vi "MH_BuffAndQDeltas.vi"(6 "queue out":refnum<queue>, 7 "DeltasBuffer":i32[](array[numeric]), 8 "erroIn":errorcluster caption="error In", 9 "WriteDelta":bool, 11 "Deltaindex":i32) -> (0 "error out":errorcluster, 1 "DeltaIndexOut":i32, 2 "DeltasBufferOut":i32[](array[numeric]))   [LabVIEW 2019]
uses:
  <userlib>/MultiHarp150/T2Lib/MH_T2DeltaQMessage.ctl
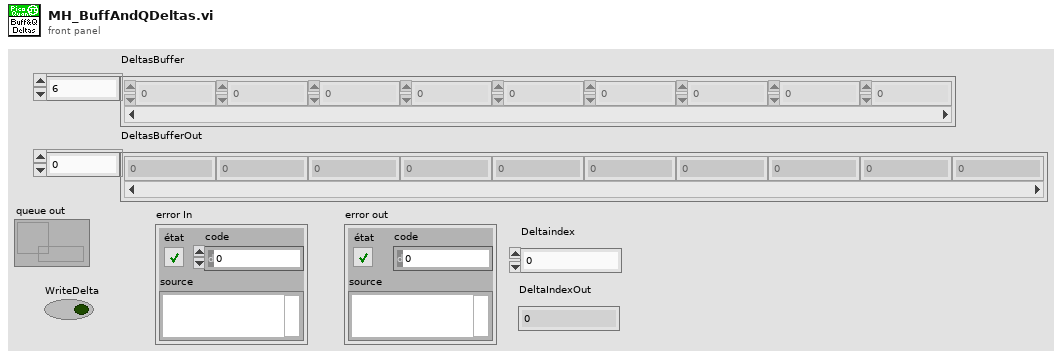
[diagram p1: front panel]
types:
  T1 = typedef "MH_T2DeltaQMessage.ctl" = cluster{"Message":string, "buffer":i32[], "Code":i32, "nactual":i32}
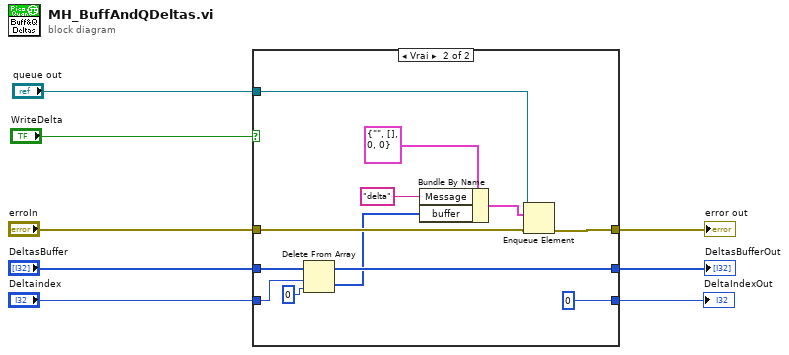
[diagram p0: block diagram]
diagram:
  n1 = case shown="Vrai" "WriteDelta" {
    tunnel: [w11 w22] -> w5
    tunnel: "erroIn" -> [w11 w21]
    tunnel: "DeltasBuffer" -> [w10 w19]
    tunnel: [w10 w19] -> w2
    tunnel: "Deltaindex" -> [w9 w18]
    tunnel: [w9 0] -> w3
    tunnel: "queue out" -> [_ w17]
    frame False {
    }
    frame True {
      n2 = Delete From Array(array=w19, length=w18, index=0 ("indice")) -> (deleted portion=w12:i32[])  [unwired: 1 out]
      n3 = Bundle By Name(cluster=T1 {"Message"="", "buffer"=[], "Code"=0, "nactual"=0} ("ClassQueue"), "Message"="delta", "buffer"=w12) -> (w13:T1)
      n4 = Enqueue Element(queue=w17, element=w13, error in (no error)=w21) -> (error out=w22:errorcluster)  [unwired: 1 in, 2 out]
    }
  }
  "DeltaIndexOut" <- w3
  "error out" <- w5
  "DeltasBufferOut" <- w2
